vi "Read Setting.vi"(8 "Error In":errorcluster) -> (0 "Error Out":errorcluster, 3 "Process Bold Characters?":bool)   [LabVIEW 2022 SP3]
doc: "This VI reads the value of the ProcessBoldCharacters setting from the \"Free Label to VI Description.ini\" file."
uses:
  <vilib>/Utility/config.llb/Read Key (Boolean).vi
  <vilib>/Utility/config.llb/NI_LVConfig.lvlib
panel:
  out "Any errors occurred inside the VI?":errorcluster
  # "Development\nControls or indicators that are useful for development or testing, but which are not outputs of the VI."
  # "Input\nInputs to the VI"
  # "Output\nOutputs of the VI"
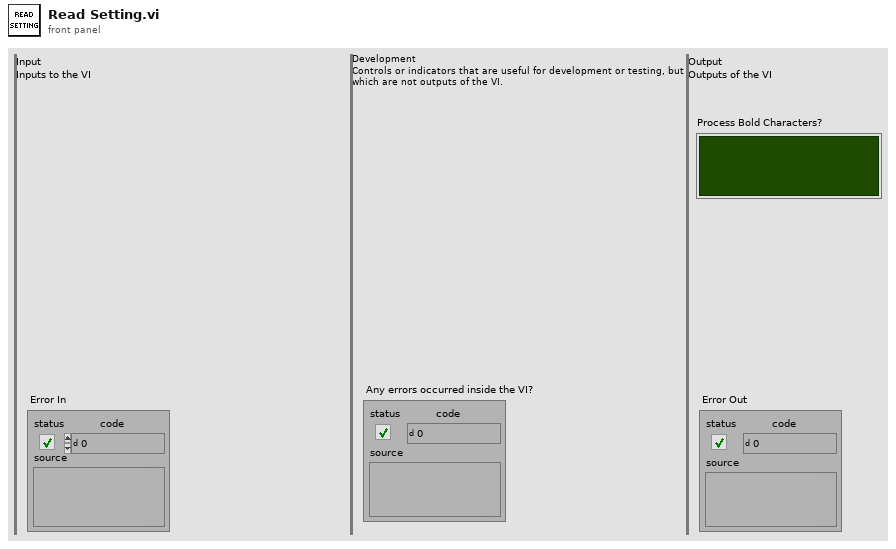
[diagram p1: front panel]
types:
  T1 = typedef "NI_LVConfig.lvlib/Config Data RefNum.ctl" = refnum<k1>
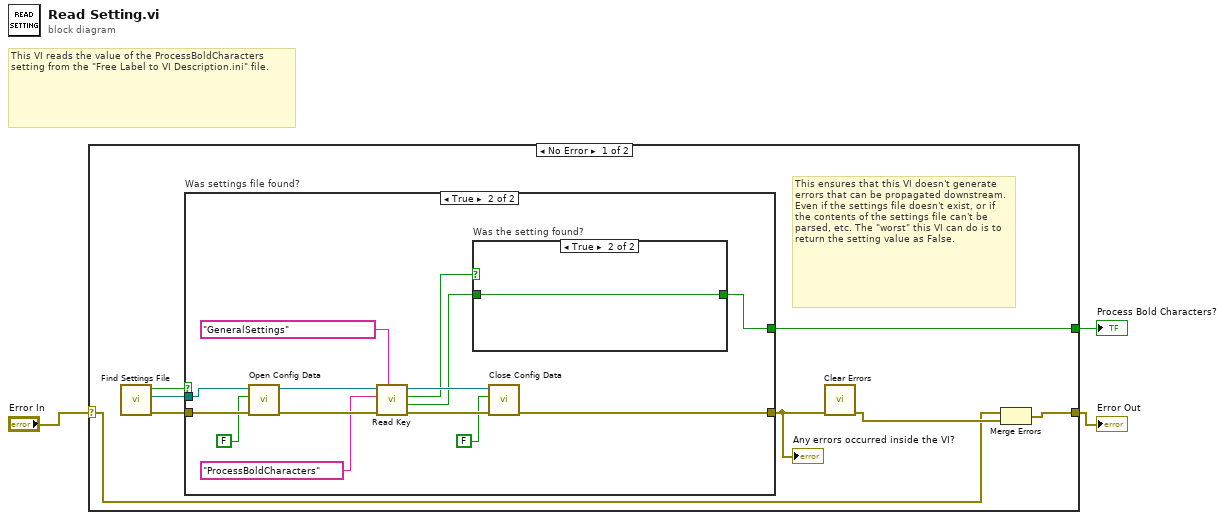
[diagram p0: block diagram]
diagram:
  # "This VI reads the value of the ProcessBoldCharacters setting from the \"Free Label to VI Description.ini\" file."
  n1 = case shown="No Error" "Error In" {
    selector: "Error In" -> [w4 w28]
    tunnel: [w6 w28] -> w2
    tunnel: [w7 _] -> w1
    frame No Error {
      # "This ensures that this VI doesn't generate errors that can be propagated downstream. Even if the settings file doesn't exist, or if the contents of the settings file can't be parsed, etc. The \"worst\" this VI can do is to return the setting value as False."
      n2 = call "Find Settings File.vi"() -> ("Error Out"=w11:errorcluster, "Settings Filepath"=w8:path, "Was settings file found?"=w9:bool)  [unwired: 9 in]
      n3 = case "Was settings file found?" shown="True" w9 {
        tunnel: w11 -> [w12 w26]
        tunnel: [w12 w20] -> w10
        tunnel: w8 -> [_ w25]
        tunnel: [_ w13] -> w7
        frame False {
          # "If the settings file (ini file)is not found behave as if the \"Process Bold Characters?\" setting is set to False."
        }
        frame True {
          n4 = call <vilib>:"Open Config Data.vi"("error in (no error)"=w26, "create file if necessary (T)"=FALSE, "configuration file path"=w25) -> ("error out"=w23:errorcluster, "refnum"=w22:T1)  [unwired: 6 in, 1 out]
          n5 = call-poly <vilib>:"Read Key.vi"("section"="GeneralSettings", "error in (no error)"=w23, "key"="ProcessBoldCharacters" ("section"), "refnum"=w22) -> ("error out"=w21:errorcluster, "value"=w14:bool, "found?"=w15:bool, "refnum out"=w19:T1)  [unwired: 4 in]
          n6 = case "Was the setting found?" shown="True" w15 {
            tunnel: w14 -> [_ w27]
            tunnel: [_ w27] -> w13
            frame False {
              # "The setting wasn't found. Behave as if the setting is set to False."
            }
            frame True {
            }
          }
          n7 = call <vilib>:"Close Config Data.vi"("error in (no error)"=w21, "write file if changed (T)"=FALSE, "refnum"=w19) -> ("error out"=w20:errorcluster)  [unwired: 7 in, 1 out]
        }
      }
      "Any errors occurred inside the VI?" <- w10
      n8 = call <vilib>:"Clear Errors.vi"("error in (no error)"=w10) -> ("error out"=w5:errorcluster)  [unwired: 5 in, 1 out]
      n9 = Merge Errors(w4, w5) -> (w6:errorcluster)
    }
    frame Error {
    }
  }
  "Error Out" <- w2
  "Process Bold Characters?" <- w1
